vi "DSet Handle to uInt32.vi"(1 "HDF5 Reference Type":T1) -> (0 "Handle":u32)   [LabVIEW 2017]
uses:
  <vilib>/UPVI/lvhdf5/reference.llb/H5R Dataset Region Ref.ctl
panel:
  # "LVHDF5 Toolkit\nCopyright (c) 2005-2013 by Jason D. Sommerville\nCopyright (c) 2014 by UPVI, LLC.\n\nThis use and distribution of this file is governed by the terms found in \nLICENSE.txt distributed with this toolkit and installed at\n <user.lib>\\_lvhdf5\\LICENSE.txt"
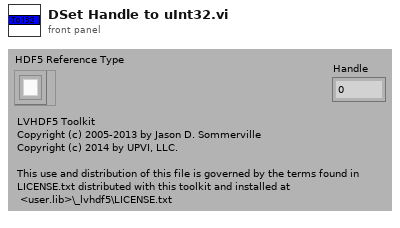
[diagram p1: front panel]
types:
  T1 = typedef "H5R Dataset Region Ref.ctl" = refnum<k1>
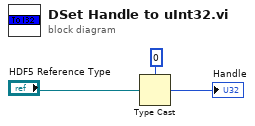
[diagram p0: block diagram]
diagram:
  n1 = Type Cast(type=u32 0, x="HDF5 Reference Type") -> (*(type *) &x=→"Handle":u32)
